vi "Read All Elements Hidden.vi"(8 "error in (no error)":errorcluster, 11 "Storage params in":refnum<class "CV-Storage.lvclass">) -> (0 "error out":errorcluster, 2 "Storage params. hidden":T1={"Storage labels"={"Original"="Original", "Corrected"="Corrected", "Binary"="Binary", "Temperature"="Temperature", "Characteristics"="Characteristics", "Mapping"="Mapping", "TemperatureValues"="TemperatureValues"}, "Characteristics headers"=["Average intensity [0-255]", "Peak intensity [0-255]", "Melt-pool size [mm²]", "Melt-pool aspect ratio []", "Melt-pool fragments []"], "CharacteristicsTemperature headers"=["Melt-pool center X [pixel]", "Melt-pool center Y [pixel]", "Orientation []"]}, 3 "Storage params out":refnum<class "CV-Storage.lvclass">)   [LabVIEW 2013, in "CameraVision.lvlib" / "CV-Storage.lvclass"]
uses:
  CV-Storage.lvclass
  Storage-parameters-advanced.ctl
  Storage-types-labels.ctl
  CV-Storage.lvclass/CV-Storage.ctl
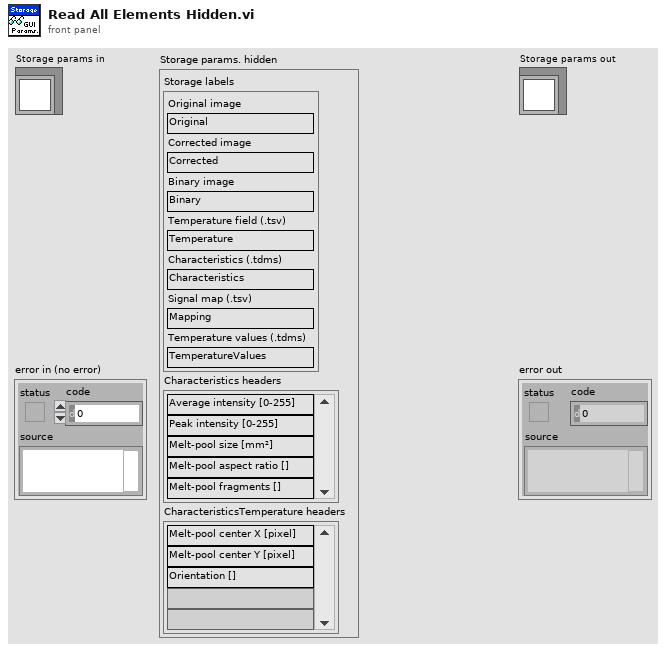
[diagram p1: front panel]
types:
  T1 = typedef "CameraVision.lvlib/CV-Storage.lvclass/Storage-parameters-advanced.ctl" = cluster{"Storage labels":T2, "Characteristics headers":string[], "CharacteristicsTemperature headers":string[]}
  T2 = typedef "CameraVision.lvlib/CV-Storage.lvclass/Storage-types-labels.ctl" = cluster{"Original":string, "Corrected":string, "Binary":string, "Temperature":string, "Characteristics":string, "Mapping":string, "TemperatureValues":string}
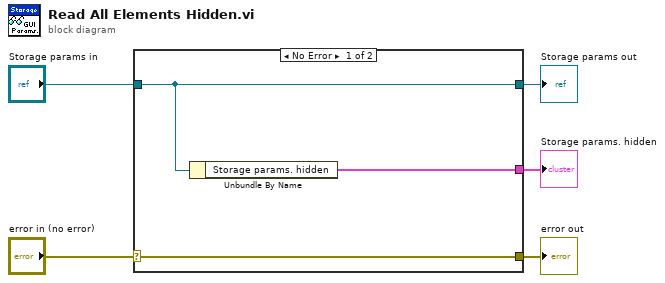
[diagram p0: block diagram]
diagram:
  n1 = case shown="No Error" "error in (no error)" {
    selector: "error in (no error)" -> [w8 w9]
    tunnel: [w8 w9] -> w4
    tunnel: [w7 w10] -> w2
    tunnel: "Storage params in" -> [w7 w10]
    tunnel: [w6 _] -> w1
    frame No Error {
      n2 = Unbundle By Name(w7) -> ("Storage params. hidden"=w6:T1)
    }
    frame Error {
    }
  }
  "error out" <- w4
  "Storage params out" <- w2
  "Storage params. hidden" <- w1
